vi "F Dwf Digital Out Counter Get.vi"(7 "pvHigh":u32, 8 "error in (no error)":errorcluster, 9 "pvLow":u32, 10 "idxChannel":i32, 11 "hdwf":i32) -> (0 "error out":errorcluster, 1 "pvLow out":u32, 3 "function return":i32, 5 "pvHigh out":u32)   [LabVIEW 2021, in "Olasdwf.lvlib"]
doc: "DWFAPI int FDwfDigitalOutCounterGet(HDWF hdwf, int idxChannel, unsigned int *pvLow, unsigned int *pvHigh);"
uses:
  Olasdwf.lvlib
  Windows/System32/dwf.dll
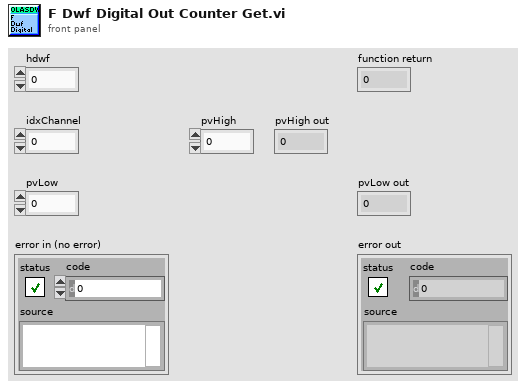
[diagram p1: front panel]
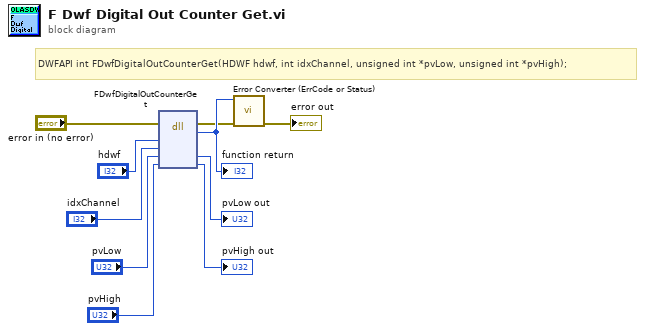
[diagram p0: block diagram]
diagram:
  # "DWFAPI int FDwfDigitalOutCounterGet(HDWF hdwf, int idxChannel, unsigned int *pvLow, unsigned int *pvHigh);"
  n1 = dll-call lib="/Windows/System32/dwf.*" fn="FDwfDigitalOutCounterGet"(error in="error in (no error)", "hdwf"="hdwf", "idxChannel"="idxChannel", "pvLow"="pvLow", "pvHigh"="pvHigh") -> (error out=w2:errorcluster, w10:i32, "pvLow"=→"pvLow out":u32, "pvHigh"=→"pvHigh out":u32)  [unwired: 4 in, 1 out]
  "function return" <- w10
  n2 = call "Error Converter (ErrCode or Status).vi"("error in (no error)"=w2, "error code"=w10) -> ("error out"=→"error out":errorcluster)  [unwired: 9 in]
